vi "GUI_MspecStitcher.vi"() -> ()   [LabVIEW 2013]
uses:
  Shared/GUI_Template/GUI_master/tcp_new_data_event.ctl
  Shared/GUI_Template/GUI_master/tcp new data cluster.ctl
panel:
  in  "MinE::1":dbl caption="Min E" min=0.0 max=0.0 format="%.1f"
  in  "DeltaE::1":dbl caption="Delta E" min=0.0 max=0.0 format="%.1f"
  in  "DeltaAngle::1":dbl caption="Delta angle" min=0.0 max=0.0 format="%.4f"
  in  "Exit":bool
  in  "MinAngle::1":dbl caption="Min angle" min=0.0 max=0.0 format="%.1f"
  in  "GUIdevice 1":string="MagSpecStitcher"
  out "tcp data event":T1
  out "error IO 2":errorcluster
  out "stitched array image":u8[][](graph)
  out "element":T2(plugin-control)
  out "error out 2":errorcluster
  out "error out":errorcluster
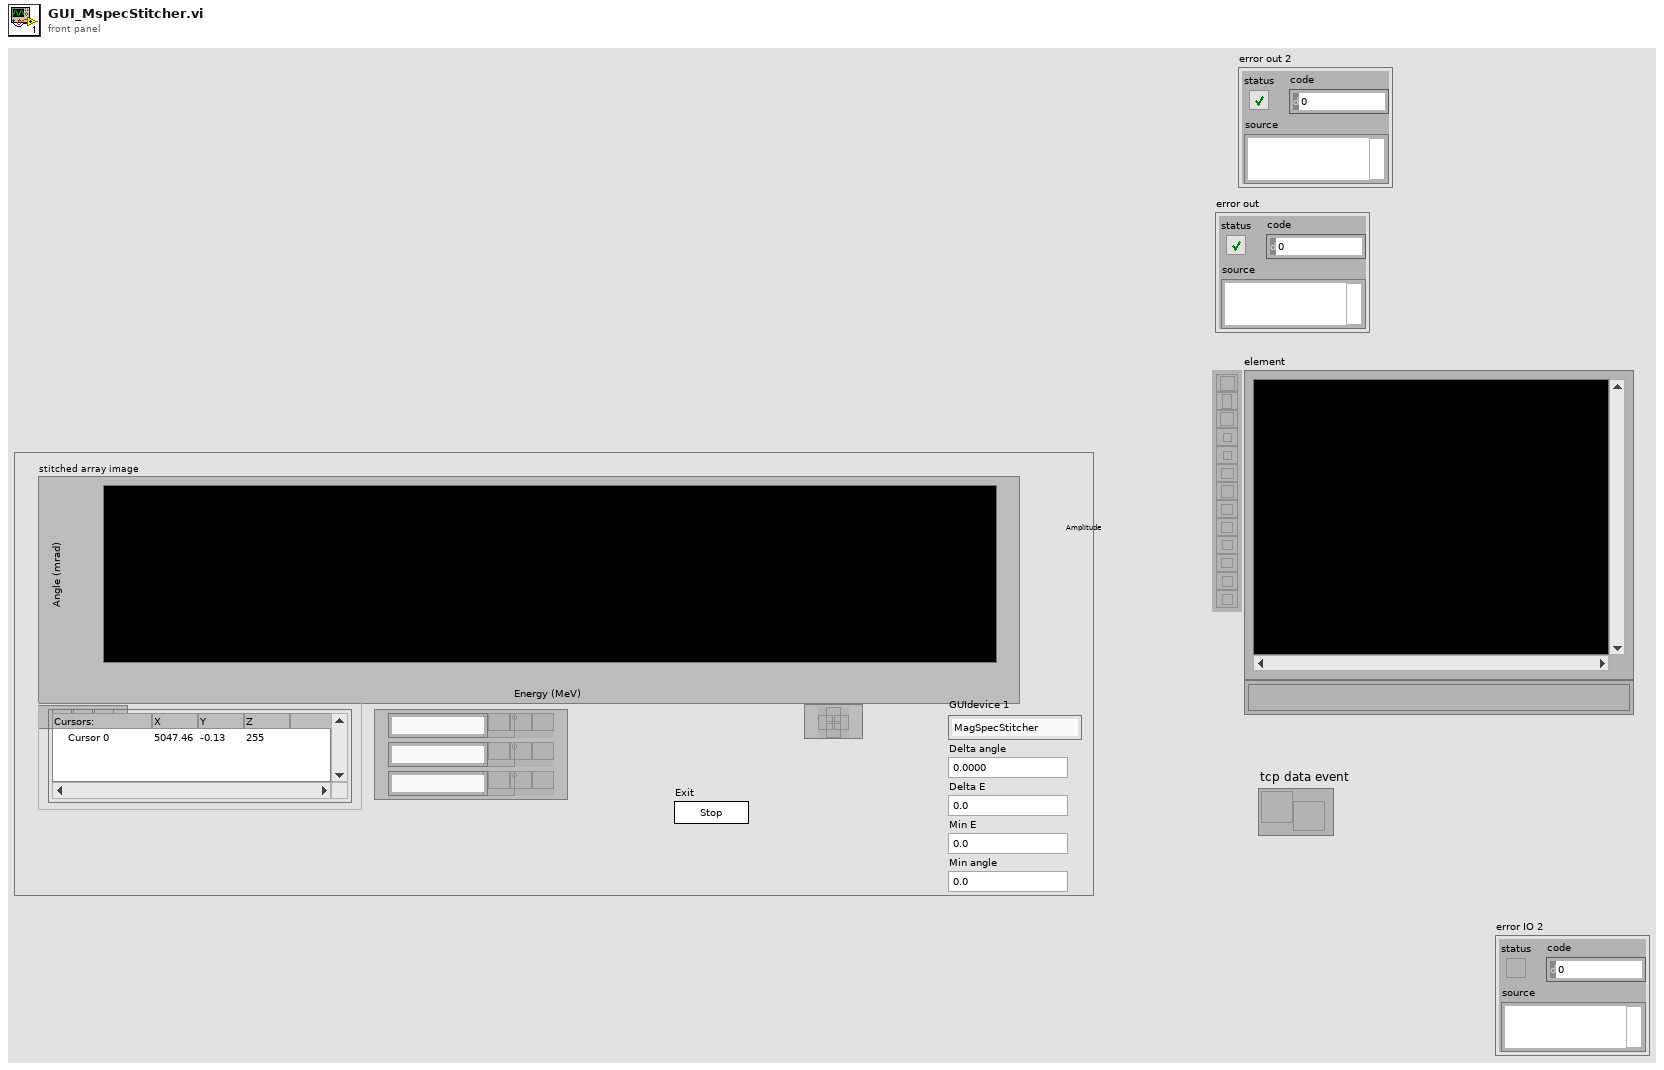
[diagram p1: front panel]
types:
  T1 = typedef "tcp_new_data_event.ctl" = refnum<user-event>
  T2 = typedef "IMAQ Image.ctl" = refnum<image>
  T3 = typedef "tcp new data cluster.ctl" = cluster{"EventEnum":enum16{"new data", "connection status update"}, "Device name":string}
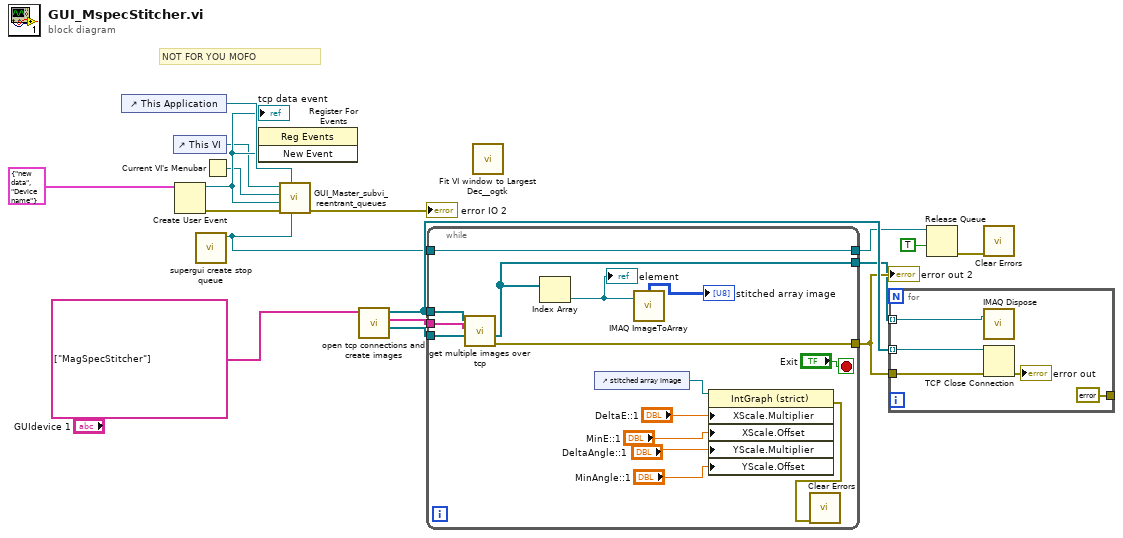
[diagram p0: block diagram]
diagram:
  # "NOT FOR YOU MOFO"
  n1 = control-ref of="This Application"() -> (w11:refnum<vi>)
  n2 = control-ref of="This VI"() -> (w5:refnum<vi>)
  n3 = Create User Event(user event datatype=T3 {"EventEnum"=enum."new data", "Device name"="Device name"} ("New Event")) -> (user event=w10:refnum<user-event>, error out=w9:errorcluster)  [unwired: 1 in]
  "tcp data event" <- w10
  n4 = call "supergui create stop queue.vi"() -> ("STOP Queue out"=w4:refnum<queue>)  [unwired: 11 in]
  n5 = Current VI's Menubar() -> (w7:refnum<k9>)
  n6 = register-events(w10) -> ()  [unwired: 2 in, 2 out]
  n7 = call "GUI_Master_subvi_reentrant_queues.vi"("STOP Queue in"=w4, "This Application"=w11, "error in (no error)"=w9, "tcp data event"=w10, "Caller menu reference"=w7, "Caller VI ref"=w5) -> ("error out"=→"error IO 2":errorcluster)  [unwired: 5 in]
  n8 = call "open tcp connections and create images.vi"("devices to get data from"=string[] ["MagSpecStitcher"]) -> ("images"=w16:T2[], "subscribe messages\nfor process vis"=w15:string[], "tcp connections"=w17:refnum<k5>[])  [unwired: 8 in]
  n9 = while {
    tunnel: w17 -> [w32]
    tunnel: w16 -> [w31]
    tunnel: w15 -> [w30]
    tunnel: [w29] -> w13
    tunnel: [w25] -> w12
    tunnel: w4 -> [w27]
    tunnel: [w27] -> w3
    stop <- "Exit" stop-if-true
    n10 = call "get multiple images over tcp.vi"("images In"=w31, "subscribeMessages"=w30, "TCP_Refs In"=w32) -> ("error out"=w29:errorcluster, "Images out"=w25:T2[])  [unwired: 4 in, 3 out]
    n11 = Index Array(array=w25) -> (element=w26:T2)  [unwired: 1 in]
    "element" <- w26
    n12 = control-ref of="stitched array image"() -> (w19:refnum<vi>)
    n13 = call "IMAQ ImageToArray"("Image"=w26) -> ("Image Pixels (U8)"=→"stitched array image":u8[][])  [unwired: 3 in, 4 out]
    n14 = property on="Property Node" class="IntGraph (strict)"(reference=w19, "XScale.Multiplier"="DeltaE::1", "XScale.Offset"="MinE::1", "YScale.Multiplier"="DeltaAngle::1", "YScale.Offset"="MinAngle::1") -> (error out=w20:errorcluster)  [unwired: 1 in, 1 out]
    n15 = call <vilib>:"Clear Errors.vi"("error in (no error)"=w20) -> ()  [unwired: 6 in, 1 out]
  }
  "error out 2" <- w13
  n16 = call <userlib>:"Fit VI window to Largest Dec__ogtk.vi"() -> ()  [unwired: 6 in, 2 out]
  n17 = for {
    tunnel: w17 -> [w37] mode=indexing
    tunnel: [errorcluster {"status"=FALSE, "code"=0, "source"=""} ("error in (no error)")] -> _
    tunnel: w13 -> [w34]
    tunnel: w12 -> [w33] mode=indexing
    n18 = call "IMAQ Dispose"("Image"=w33) -> ()  [unwired: 5 in, 1 out]
    n19 = TCP Close Connection(connection ID=w37, error in (no error)=w34) -> (error out=→"error out":errorcluster)  [unwired: 1 in, 1 out]
  }
  n20 = Release Queue(queue=w3, force destroy? (F)=TRUE) -> (error out=w1:errorcluster)  [unwired: 1 in, 2 out]
  n21 = call <vilib>:"Clear Errors.vi"("error in (no error)"=w1) -> ()  [unwired: 6 in, 1 out]
